vi "Trajectory_Execution_Execute_Reverse_W_PoseEst.vi"(5 "Effective Track Width FT":dbl, 7 "Max Speed\nFT/SEC":dbl, 8 "Init":bool, 11 "Input Sensors":T4) -> (0 "AtReference":bool, 1 "Right Speed Target":dbl, 2 "Left Speed Target":dbl, 3 "outRAMSETE (SI)":T6={"B"=2.0, "Zeta"=0.7, "poseTolerance"={"TRANSLATION"={"X"=0.0, "Y"=0.0}, "ROTATION"={"VALUE"=0.0, "COS"=1.0, "SIN"=0.0}}, "poseError"={"TRANSLATION"={"X"=0.0, "Y"=0.0}, "ROTATION"={"VALUE"=0.0, "COS"=1.0, "SIN"=0.0}}, "Enabled"=TRUE} {"poseError"."ROTATION"."SIN" format="%13.4f"; "poseError"."ROTATION"."COS" format="%13.4f"; "poseError"."ROTATION"."VALUE" format="%13.4f"; "poseError"."TRANSLATION"."Y" format="%14.3f"; "poseError"."TRANSLATION"."X" format="%14.3f"; "poseTolerance"."ROTATION"."SIN" format="%13.4f"; "poseTolerance"."ROTATION"."COS" format="%13.4f"; "poseTolerance"."ROTATION"."VALUE" format="%13.4f"; "poseTolerance"."TRANSLATION"."Y" format="%14.3f"; "poseTolerance"."TRANSLATION"."X" format="%14.3f"; "Zeta" format="%12.3f"; "B" format="%12.3f"}, 4 "OutputTRAJ_STATE (SI)":T5={"TimeSeconds"=0.0, "Velocity"=0.0, "Acceleration"=0.0, "POSE"={"TRANSLATION"={"X"=0.0, "Y"=0.0}, "ROTATION"={"VALUE"=0.0, "COS"=1.0, "SIN"=0.0}}, "Curvature"=0.0} {"POSE"."ROTATION"."SIN" format="%13.4f"; "POSE"."ROTATION"."COS" format="%13.4f"; "POSE"."ROTATION"."VALUE" format="%13.4f"; "POSE"."TRANSLATION"."Y" format="%14.3f"; "POSE"."TRANSLATION"."X" format="%14.3f"})   [LabVIEW 2019]
uses:
  <vilib>/Rock Robotics/WPI/ThirdParty/JAS_Junk/TrajLib/TypeDef/RAMSETE.ctl
  <vilib>/Rock Robotics/WPI/ThirdParty/JAS_Junk/TrajLib/TypeDef/POSE2D.ctl
  <vilib>/Rock Robotics/WPI/ThirdParty/JAS_Junk/TrajLib/TypeDef/TRANSLATION2D.ctl
  <vilib>/Rock Robotics/WPI/ThirdParty/JAS_Junk/TrajLib/TypeDef/ROTATION2D.ctl
  <vilib>/Rock Robotics/WPI/ThirdParty/JAS_Junk/TrajLib/TypeDef/TRAJ_STATE.ctl
  Trajectory_Execution_Sensors.ctl
  <vilib>/Rock Robotics/WPI/ThirdParty/JAS_Junk/TrajLib/Rotation2d_CreateAngle.vi
  <vilib>/Rock Robotics/SystemInterfaces/NetworkCommunication/NetComm_UsageReport_report.vi
  <vilib>/Rock Robotics/WPI/ThirdParty/JAS_Junk/TrajLib/Translation2d_Create.vi
  <vilib>/Rock Robotics/WPI/ThirdParty/JAS_Junk/TrajLib/Conv_POSE2D_SI_Eng.vi
  <vilib>/Rock Robotics/WPI/ThirdParty/JAS_Junk/TrajLib/Conv_Radians_Deg.vi
  Trajectory_Execution_Globals.vi
  <vilib>/Rock Robotics/WPI/ThirdParty/JAS_Junk/TrajLib/Util_LibraryGlobals.vi
  <vilib>/Rock Robotics/WPI/ThirdParty/JAS_Junk/TrajLib/Trajectory_Library.lvlib
panel:
  out "Pose Est Info":cluster{"Estimated Pose":T1, "Error":bool} {"Estimated Pose"."ROTATION"."SIN" format="%13.4f"; "Estimated Pose"."ROTATION"."COS" format="%13.4f"; "Estimated Pose"."ROTATION"."VALUE" format="%13.4f"; "Estimated Pose"."TRANSLATION"."Y" format="%14.3f"; "Estimated Pose"."TRANSLATION"."X" format="%14.3f"}
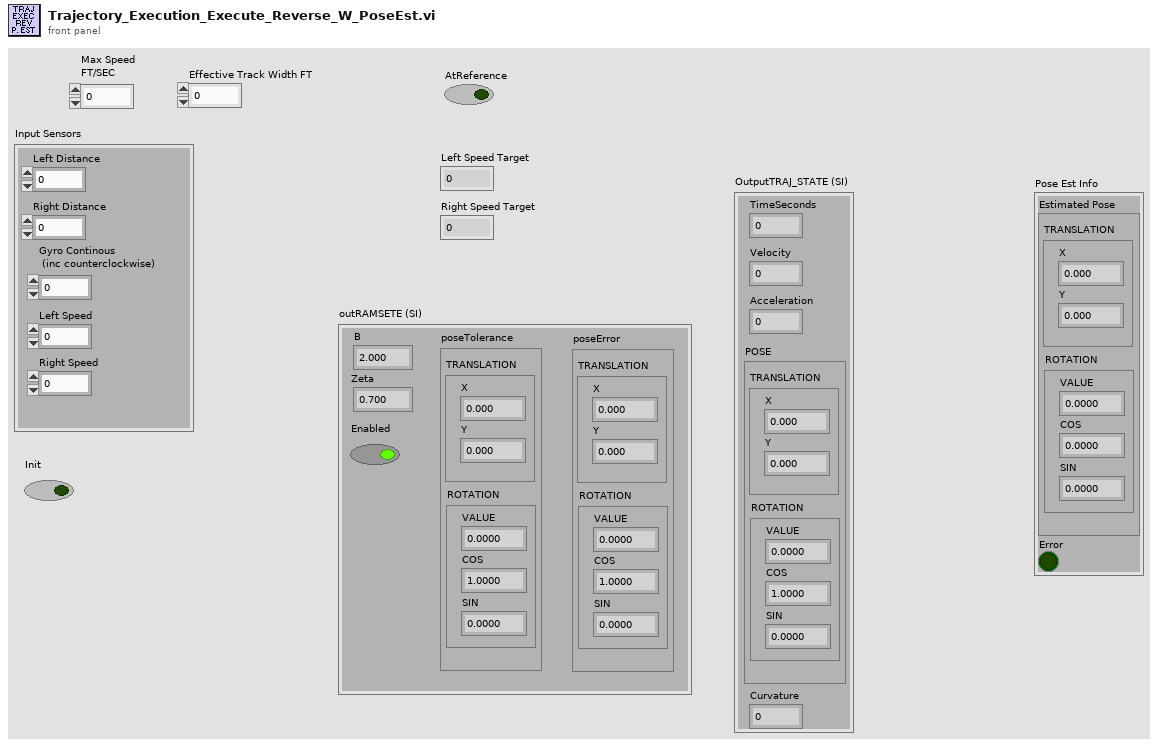
[diagram p1: front panel]
types:
  T1 = typedef "Trajectory_Library.lvlib/POSE2D.ctl" = cluster{"TRANSLATION":T2, "ROTATION":T3}
  T2 = typedef "Trajectory_Library.lvlib/TRANSLATION2D.ctl" = cluster{"X":dbl, "Y":dbl}
  T3 = typedef "Trajectory_Library.lvlib/ROTATION2D.ctl" = cluster{"VALUE":dbl, "COS":dbl, "SIN":dbl}
  T4 = typedef "Trajectory_Execution_Sensors.ctl" = cluster{"Left Distance":dbl, "Right Distance":dbl, "Gyro Continous\n (inc counterclockwise)":dbl, "Left Speed":dbl, "Right Speed":dbl}
  T5 = typedef "Trajectory_Library.lvlib/TRAJ_STATE.ctl" = cluster{"TimeSeconds":dbl, "Velocity":dbl, "Acceleration":dbl, "POSE":T1, "Curvature":dbl}
  T6 = typedef "Trajectory_Library.lvlib/RAMSETE.ctl" = cluster{"B":dbl, "Zeta":dbl, "poseTolerance":T1, "poseError":T1, "Enabled":bool}
  T7 = typedef "Trajectory_Library.lvlib/DIFF_DRIVE_POSE_EST.ctl" = cluster{"M_VisionContR":T8, "m_nominal_dT":dbl, "m_PrevTime_Sec":dbl, "m_GyroOffset":T3, "m_PrevAngle":T3, "StartLeftEnc_M":dbl, "StartRightEnc_M":dbl, "m_Observer":T9, "Pose_Buffer":T12}
  T8 = typedef "NI_Matrix.lvlib/RealMatrix.ctl" = dbl[][]
  T9 = typedef "Trajectory_Library.lvlib/UNSCENTED_KALMAN_FILTER.ctl" = cluster{"m_P":T8, "m_xHat":T8, "States":i32, "Outputs":i32, "m_ContR":T8, "m_ContQ":T8, "m_SigmasF":T8, "m_dT_Sec":dbl, "MERWE_SCALED_SIGMA_PTS":T10, "meanFuncX":T11, "meanFuncY":T11, "residualFuncX":T11, "residualFuncY":T11, "addFuncX":T11, "addFuncXExtra":variant, "residualFuncYExtra":variant, "residualFuncXExtra":variant, "MeanFuncYExtra":variant, "MeanFuncXExtra":variant, "Inputs":i32}
  T10 = typedef "Trajectory_Library.lvlib/MERWE_SCALED_SIGMA_PTS.ctl" = cluster{"m_Wm":T8, "States":i32, "Alpha":dbl, "m_Wc":T8, "Kappa":i32}
  T11 = typedef "Trajectory_Library.lvlib/CALLBACK_FUNC_TYPE.ctl" = refnum<vi>
  T12 = typedef "Trajectory_Library.lvlib/TIME_INTERPOLATABLE_POSE2D.ctl" = cluster{"TimeStamps":dbl[], "Pose":T1[], "Min_TimeStamp":dbl, "Max_TimeStamp":dbl, "ItemCount":i32, "MaxBufferTime":dbl}
  T13 = typedef "Trajectory_Library.lvlib/TRAJECTORY.ctl" = cluster{"TotalTImeSecs":dbl, "States":T5[]}
  T14 = typedef "Trajectory_Library.lvlib/DIFF_DRIVE_KINEMATICS.ctl" = cluster{"TrackWidth_Meters":dbl}
  T15 = typedef "Trajectory_Library.lvlib/CHASSIS_SPEEDS.ctl" = cluster{"vX":dbl, "vY":dbl, "vOmega":dbl}
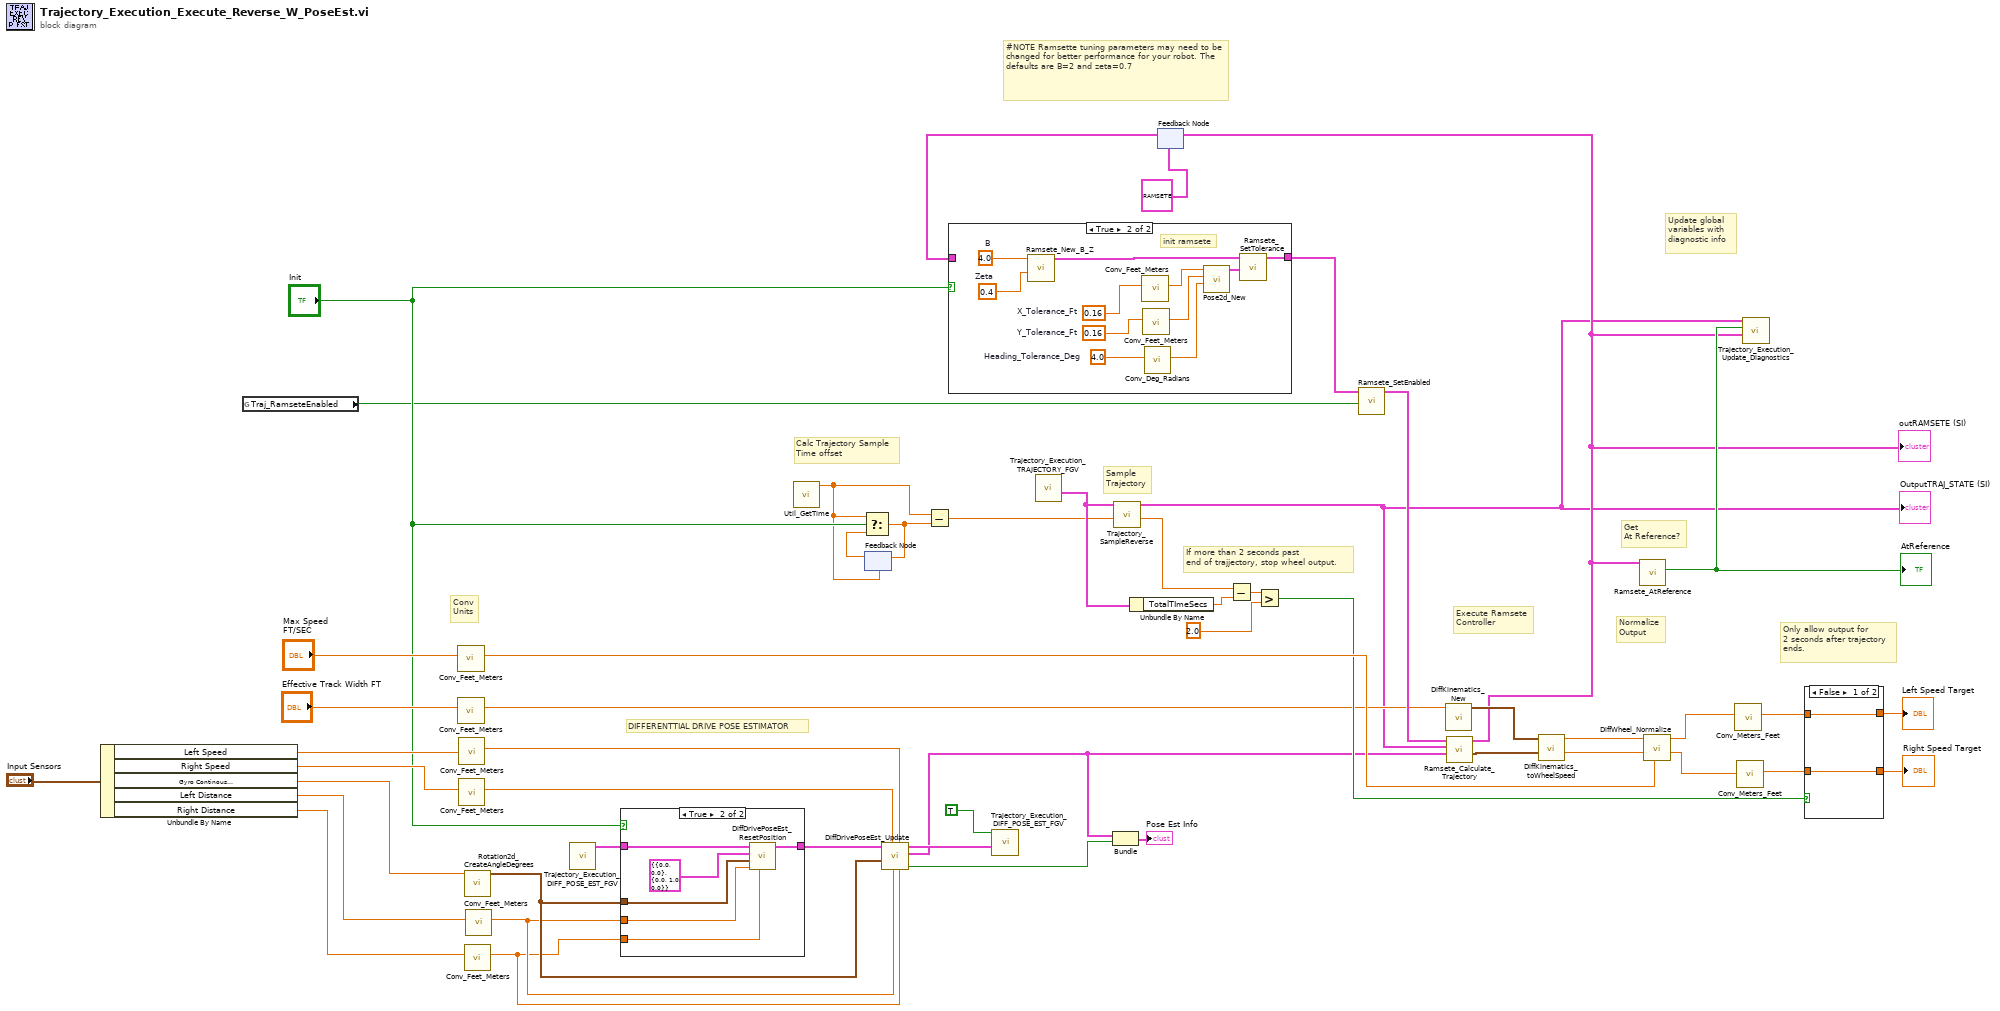
[diagram p0: block diagram]
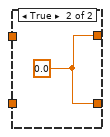
[diagram p4: hidden frame]
diagram:
  # "Get \nAt Reference?"
  # "Conv\nUnits"
  # "Calc Trajectory Sample\nTime offset"
  # "If more than 2 seconds past\nend of trajjectory, stop wheel output."
  # "Normalize\nOutput"
  # "Execute Ramsete\nController"
  # "Update global\nvariables with\ndiagnostic info"
  # "Sample\nTrajectory"
  # "DIFFERENTTIAL DRIVE POSE ESTIMATOR"
  # "#NOTE Ramsette tuning parameters may need to be changed for better performance for your robot. The defaults are B=2 and zeta=0.7"
  # "Only allow output for\n2 seconds after trajectory\nends."
  n1 = Unbundle By Name("Input Sensors") -> ("Left Speed"=w26:dbl, "Right Speed"=w25:dbl, "Gyro Continous\n (inc counterclockwise)"=w5:dbl, "Left Distance"=w4:dbl, "Right Distance"=w3:dbl)
  n2 = global read "Trajectory_Execution_Globals.vi" "Traj_RamseteEnabled"() -> (w2:bool)
  n3 = call <vilib>:"Conv_Feet_Meters.vi"("Feet"="Max Speed\nFT/SEC") -> ("Meters"=w48:dbl)  [unwired: 10 in]
  n4 = call <vilib>:"Conv_Feet_Meters.vi"("Feet"="Effective Track Width FT") -> ("Meters"=w10:dbl)  [unwired: 10 in]
  n5 = call <vilib>:"Conv_Feet_Meters.vi"("Feet"=w26) -> ("Meters"=w24:dbl)  [unwired: 10 in]
  n6 = call <vilib>:"Conv_Feet_Meters.vi"("Feet"=w25) -> ("Meters"=w23:dbl)  [unwired: 10 in]
  n7 = call <vilib>:"Rotation2d_CreateAngleDegrees.vi"("Angle_Degrees"=w5) -> ("ROTATION"=w29:T3)  [unwired: 10 in]
  n8 = call <vilib>:"Conv_Feet_Meters.vi"("Feet"=w3) -> ("Meters"=w22:dbl)  [unwired: 10 in]
  n9 = call <vilib>:"Conv_Feet_Meters.vi"("Feet"=w4) -> ("Meters"=w27:dbl)  [unwired: 10 in]
  n10 = call "Trajectory_Execution_DIFF_POSE_EST_FGV.vi"() -> ("out DIFF_DRIVE_POSE_EST 2"=w32:T7)  [unwired: 11 in]
  n11 = case shown="True" "Init" {
    tunnel: w32 -> [w51 w57]
    tunnel: [w51 w56] -> w31
    tunnel: w27 -> [_ w55]
    tunnel: w22 -> [_ w54]
    tunnel: w29 -> [_ w52]
    frame False {
    }
    frame True {
      n12 = call <vilib>:"DiffDrivePoseEst_ResetPosition.vi"("RightDistance_M"=w54, "LeftDistance_M"=w55, "Gyro"=w52, "Pose"=T1 {"TRANSLATION"={"X"=0.0, "Y"=0.0}, "ROTATION"={"VALUE"=0.0, "COS"=1.0, "SIN"=0.0}}, "in DiffDrivePoseEstimate"=w57) -> ("Out DiffDrivePoseEstimate"=w56:T7)  [unwired: 6 in]
    }
  }
  n13 = call <vilib>:"Util_GetTime.vi"() -> ("FPGA_Time_Seconds"=w1:dbl)  [unwired: 10 in, 1 out]
  n14 = feedback #1(w1) -> (w7:dbl)
  n15 = Select(t=w1, s="Init", f=w7) -> (s? t:f=w8:dbl)
  n16 = feedback-in #1(w8) -> ()
  n17 = call <vilib>:"DiffDrivePoseEst_Update.vi"("RightDistance"=w22, "LeftSpeed"=w24, "LeftDistance"=w27, "RightSpeed"=w23, "GyroAngle"=w29, "in DiffDrivePoseEstimate"=w31) -> ("Error"=w21:bool, "Estimated Pose"=w11:T1, "Out DiffDrivePoseEstimate"=w30:T7)  [unwired: 3 in]
  n18 = Subtract(x=w1, y=w8) -> (x-y=w43:dbl)
  n19 = call "Trajectory_Execution_DIFF_POSE_EST_FGV.vi"("IN DIFF_DRIVE_POSE_EST"=w30, "WRITE"=TRUE) -> ()  [unwired: 9 in, 1 out]
  n20 = call "Trajectory_Execution_TRAJECTORY_FGV.vi"() -> ("outTRAJECTORY"=w45:T13)  [unwired: 11 in]
  n21 = Bundle("Estimated Pose"=w11, "Error"=w21) -> (→"Pose Est Info":cluster{"Estimated Pose":T1, "Error":bool})  [unwired: 1 in]
  n22 = call <vilib>:"Trajectory_SampleReverse.vi"("Time"=w43, "InputTRAJECTORY"=w45) -> ("OutputTRAJ_STATE"=w9:T5)  [unwired: 9 in]
  "OutputTRAJ_STATE (SI)" <- w9
  n23 = Unbundle By Name(w45) -> ("TotalTImeSecs"=w44:dbl)
  n24 = feedback #2(T6 {"B"=2.0, "Zeta"=0.7, "poseTolerance"={"TRANSLATION"={"X"=0.0, "Y"=0.0}, "ROTATION"={"VALUE"=0.0, "COS"=1.0, "SIN"=0.0}}, "poseError"={"TRANSLATION"={"X"=0.0, "Y"=0.0}, "ROTATION"={"VALUE"=0.0, "COS"=1.0, "SIN"=0.0}}, "Enabled"=TRUE} ("RAMSETE")) -> (w35:T6)
  n25 = case shown="True" "Init" {
    tunnel: w35 -> [w58 _]
    tunnel: [w58 w65] -> w19
    frame False {
    }
    frame True {
      w66 = 0.4  # Zeta
      w67 = 4.0  # B
      w61 = 4.0  # Heading_Tolerance_Deg
      w59 = 0.16  # Y_Tolerance_Ft
      w60 = 0.16  # X_Tolerance_Ft
      # "init ramsete"
      n26 = call <vilib>:"Ramsete_New_B_Z.vi"("Zeta"=w66, "B"=w67) -> ("outRAMSETE"=w69:T6)  [unwired: 9 in]
      n27 = call <vilib>:"Conv_Feet_Meters.vi"("Feet"=w60) -> ("Meters"=w64:dbl)  [unwired: 10 in]
      n28 = call <vilib>:"Conv_Feet_Meters.vi"("Feet"=w59) -> ("Meters"=w63:dbl)  [unwired: 10 in]
      n29 = call <vilib>:"Conv_Deg_Radians.vi"("Degress"=w61) -> ("Radians"=w62:dbl)  [unwired: 10 in]
      n30 = call <vilib>:"Pose2d_New.vi"("Heading"=w62, "Y"=w63, "X"=w64) -> ("out POSe"=w68:T1)  [unwired: 8 in]
      n31 = call <vilib>:"Ramsete_SetTolerance.vi"("tolerancePose"=w68, "inRAMSETE"=w69) -> ("outRAMSETE"=w65:T6)  [unwired: 9 in]
    }
  }
  n32 = Subtract(x=w43, y=w44) -> (x-y=w42:dbl)
  n33 = Greater?(x=w42, y=2.0) -> (0:w40:bool)
  n34 = call <vilib>:"Ramsete_SetEnabled.vi"("Enabled"=w2, "inRAMSETE"=w19) -> ("outRAMSETE"=w12:T6)  [unwired: 9 in]
  n35 = call <vilib>:"DiffKinematics_New.vi"("TrackWidth_Meters"=w10) -> ("DIFF_DRIVE_KINEMATICS"=w18:T14)  [unwired: 10 in]
  n36 = call <vilib>:"Ramsete_Calculate_Trajectory.vi"("CurrentPOSE"=w11, "TRAJ_STATE"=w9, "inRAMSETE"=w12) -> ("CHASSIS Speeds"=w17:T15, "outRAMSETE"=w13:T6)  [unwired: 7 in]
  "outRAMSETE (SI)" <- w13
  n37 = feedback-in #2(w13) -> ()
  n38 = call <vilib>:"DiffKinematics_toWheelSpeed.vi"("CHASSIS Speed"=w17, "DIFF_DRIVE_KINEMATICS"=w18) -> ("RightVelocity"=w15:dbl, "LeftVelocity"=w16:dbl)  [unwired: 8 in]
  n39 = call <vilib>:"Ramsete_AtReference.vi"("RAMSETE"=w13) -> ("AtReference"=w14:bool)  [unwired: 10 in]
  "AtReference" <- w14
  n40 = call <vilib>:"DiffWheel_Normalize.vi"("Max Speed"=w48, "Right Wheel Demand"=w15, "Left Wheel Demand"=w16) -> ("Normalized Right Wheel Demand"=w46:dbl, "Normalized Left Wheel Demand"=w47:dbl)  [unwired: 7 in]
  n41 = call <vilib>:"Conv_Meters_Feet.vi"("Meters"=w47) -> ("Feet"=w37:dbl)  [unwired: 10 in]
  n42 = call <vilib>:"Conv_Meters_Feet.vi"("Meters"=w46) -> ("Feet"=w36:dbl)  [unwired: 10 in]
  n43 = call "Trajectory_Execution_Update_Diagnostics.vi"("outRAMSETE (SI)"=w13, "AtReference"=w14, "OutputTRAJ_STATE (SI)"=w9) -> ()  [unwired: 9 in]
  n44 = case shown="False" w40 {
    tunnel: [w71 w72] -> w39
    tunnel: [w70 w72] -> w38
    tunnel: w37 -> [w71 _]
    tunnel: w36 -> [w70 _]
    frame False {
    }
    frame True {
      w72 = 0.0
    }
  }
  "Left Speed Target" <- w39
  "Right Speed Target" <- w38
